vi "LPC query speak rate.vi"(8 "error in (no error)":errorcluster, 11 "VISA resource name":refnum<visa-resource-name>="GPIB0::8::INSTR") -> (0 "error out":errorcluster, 2 "speak rate":dbl, 3 "VISA resource name out":refnum<visa-resource-name>)   [LabVIEW 2009, in "Laser Power Controller.lvclass"]
doc: "Reads the speak rate of the LPC (laser power controller). This controls the rate at which the LPC sends back log entries. The speak rate should be set to zero while issuing commands or performing queries, to avoid reading a log entry when another response was expected."
uses:
  Laser Power Controller.lvclass
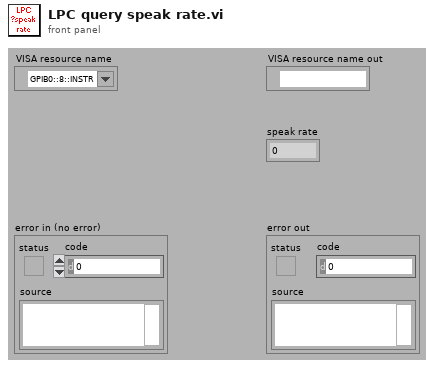
[diagram p1: front panel]
types:
  T1 = typedef "Semaphore RefNum" = refnum<k1>
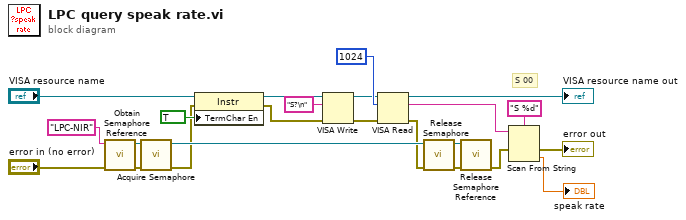
[diagram p0: block diagram]
diagram:
  # "S 00"
  n1 = call <vilib>:"Obtain Semaphore Reference.vi"("error in (no error)"="error in (no error)", "name (unnamed)"="LPC-NIR") -> ("error out"=w21:errorcluster, "semaphore"=w20:T1)  [unwired: 1 in, 3 out]
  n2 = call <vilib>:"Acquire Semaphore.vi"("error in (no error)"=w21, "semaphore"=w20) -> ("error out"=w12:errorcluster, "semaphore out"=w17:T1)  [unwired: 1 in, 3 out]
  n3 = property class="Instr"(reference="VISA resource name", error in=w12, "TermChar En"=TRUE ("Message Based Settings:Termination Character Enable")) -> (error out=w11:errorcluster)  [unwired: 1 out]
  n4 = VISA Write(VISA resource name="VISA resource name", write buffer="S?\n", error in (no error)=w11) -> (VISA resource name out=w7:refnum<visa-resource-name>, error out=w8:errorcluster)  [unwired: 1 out]
  n5 = VISA Read(VISA resource name=w7, byte count=u32 1024, error in (no error)=w8) -> (VISA resource name out=→"VISA resource name out":refnum<visa-resource-name>, read buffer=w4:string, error out=w9:errorcluster)  [unwired: 1 out]
  n6 = call <vilib>:"Release Semaphore.vi"("error in (no error)"=w9, "semaphore"=w17) -> ("error out"=w19:errorcluster, "semaphore out"=w18:T1)  [unwired: 4 out]
  n7 = call <vilib>:"Release Semaphore Reference.vi"("error in (no error)"=w19, "semaphore"=w18) -> ("error out"=w3:errorcluster)  [unwired: 9 out]
  n8 = Scan From String(format string="S %d", input string=w4, error in=w3) -> (error out=→"error out":errorcluster, output 1=→"speak rate":dbl)  [unwired: 1 in, 3 out]
